vi "Read Parameters.vi"(4 "error in (no error)":errorcluster, 7 "appended path":path) -> (0 "error out":errorcluster, 3 "rangeParams":T1)   [LabVIEW 2015]
uses:
  <vilib>/Utility/config.llb/Read Key (Double).vi
  <vilib>/Utility/config.llb/NI_LVConfig.lvlib
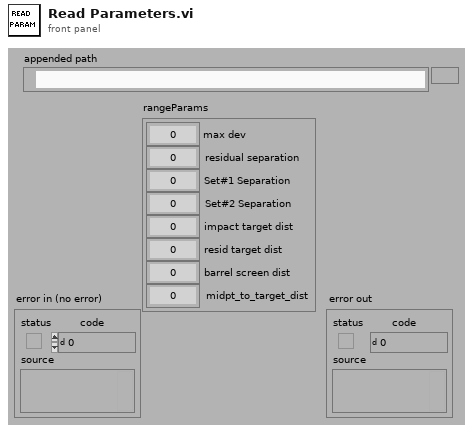
[diagram p1: front panel]
types:
  T1 = cluster{"max dev":sgl, "residual separation":sgl, "Set#1 Separation":sgl, "Set#2 Separation ":sgl, "impact target dist":sgl, "resid target dist":sgl, "barrel screen dist":sgl, "midpt_to_target_dist":sgl}
  T2 = typedef "NI_LVConfig.lvlib/Config Data RefNum.ctl" = refnum<k1>
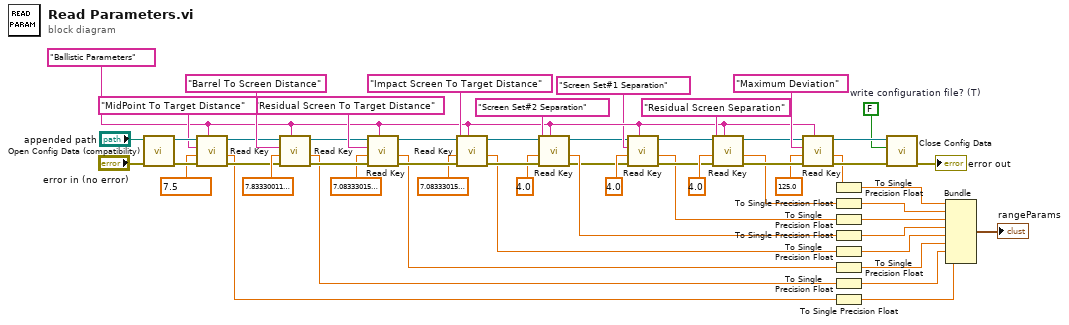
[diagram p0: block diagram]
diagram:
  w36 = FALSE  # write configuration file? (T)
  w8 = "Ballistic Parameters"
  n1 = call <vilib>:"Open Config Data (compatibility).vi"("error in (no error)"="error in (no error)", "configuration file path"="appended path") -> ("error out"=w27:errorcluster, "refnum"=w25:T2)  [unwired: 7 in, 1 out]
  n2 = call-poly <vilib>:"Read Key.vi"("section"=w8, "error in (no error)"=w27, "default value"=7.5, "key"="MidPoint To Target Distance", "refnum"=w25) -> ("error out"=w26:errorcluster, "value"=w22:dbl, "refnum out"=w24:T2)  [unwired: 4 out]
  n3 = call-poly <vilib>:"Read Key.vi"("section"=w8, "error in (no error)"=w26, "default value"=7.8333001136779785, "key"="Barrel To Screen Distance", "refnum"=w24) -> ("error out"=w52:errorcluster, "value"=w37:dbl, "refnum out"=w44:T2)  [unwired: 4 out]
  n4 = call-poly <vilib>:"Read Key.vi"("section"=w8, "error in (no error)"=w52, "default value"=7.083330154418945, "key"="Residual Screen To Target Distance", "refnum"=w44) -> ("error out"=w48:errorcluster, "value"=w39:dbl, "refnum out"=w43:T2)  [unwired: 4 out]
  n5 = call-poly <vilib>:"Read Key.vi"("section"=w8, "error in (no error)"=w48, "default value"=7.083330154418945, "key"="Impact Screen To Target Distance", "refnum"=w43) -> ("error out"=w49:errorcluster, "value"=w38:dbl, "refnum out"=w42:T2)  [unwired: 4 out]
  n6 = call-poly <vilib>:"Read Key.vi"("section"=w8, "error in (no error)"=w49, "default value"=4.0, "key"="Screen Set#2 Separation", "refnum"=w42) -> ("error out"=w4:errorcluster, "value"=w40:dbl, "refnum out"=w6:T2)  [unwired: 4 out]
  n7 = call-poly <vilib>:"Read Key.vi"("section"=w8, "error in (no error)"=w4, "default value"=4.0, "key"="Screen Set#1 Separation", "refnum"=w6) -> ("error out"=w3:errorcluster, "value"=w2:dbl, "refnum out"=w5:T2)  [unwired: 4 out]
  n8 = call-poly <vilib>:"Read Key.vi"("section"=w8, "error in (no error)"=w3, "default value"=4.0, "key"="Residual Screen Separation", "refnum"=w5) -> ("error out"=w50:errorcluster, "value"=w46:dbl, "refnum out"=w41:T2)  [unwired: 4 out]
  n9 = call-poly <vilib>:"Read Key.vi"("section"=w8, "error in (no error)"=w50, "default value"=125.0, "key"="Maximum Deviation", "refnum"=w41) -> ("error out"=w51:errorcluster, "value"=w47:dbl, "refnum out"=w45:T2)  [unwired: 4 out]
  n10 = To Single Precision Float(number=w47) -> (single precision float=w18:sgl)
  n11 = To Single Precision Float(number=w46) -> (single precision float=w17:sgl)
  n12 = To Single Precision Float(number=w2) -> (single precision float=w1:sgl)
  n13 = To Single Precision Float(number=w40) -> (single precision float=w16:sgl)
  n14 = To Single Precision Float(number=w38) -> (single precision float=w14:sgl)
  n15 = To Single Precision Float(number=w39) -> (single precision float=w13:sgl)
  n16 = To Single Precision Float(number=w37) -> (single precision float=w12:sgl)
  n17 = To Single Precision Float(number=w22) -> (single precision float=w11:sgl)
  n18 = call <vilib>:"Close Config Data.vi"("error in (no error)"=w51, "write file if changed (T)"=w36, "refnum"=w45) -> ("error out"=→"error out":errorcluster)  [unwired: 8 out]
  n19 = Bundle(w18, w17, w1, w16, w14, w13, w12, w11) -> (→"rangeParams":cluster{sgl, sgl, sgl, sgl, sgl, sgl, sgl, sgl})  [unwired: 1 out]
